vi "Check VI_EXE_Exit wo Confirmation.vi"(8 "error in":errorcluster) -> (0 "error out":errorcluster)   [LabVIEW 2018]
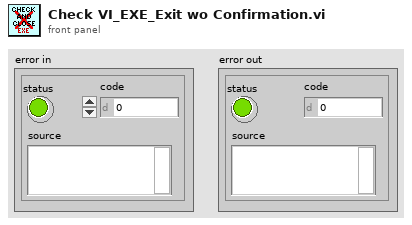
[diagram p1: front panel]
types:
  T1 = enum32{"invalid app kind", "Development System", "Run Time System", "Student Edition", "Embedded LabVIEW", "Evaluation", "Custom"}
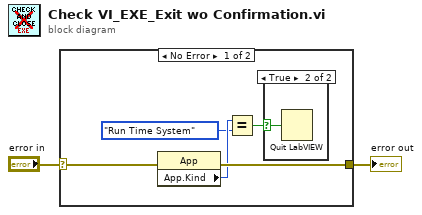
[diagram p0: block diagram]
diagram:
  n1 = case shown="No Error" "error in" {
    selector: "error in" -> [w3 w9]
    tunnel: [w7 w9] -> w2
    frame No Error {
      n2 = property class="App"(error in=w3) -> (error out=w7:errorcluster, "App.Kind"=w6:T1)  [unwired: 1 in, 1 out]
      n3 = Equal?(x=w6, y=T1."Run Time System") -> (x = y?=w4:bool)
      n4 = case shown="True" w4 {
        selector: w4 -> [_ w8]
        frame False {
        }
        frame True {
          n5 = Quit LabVIEW(quit? (T)=w8) -> ()
        }
      }
    }
    frame Error {
    }
  }
  "error out" <- w2
